vi "Get Users.vi"(8 "error in (no error)":errorcluster, 11 "Data.PG":refnum<class "Data.PGSQL.lvclass">) -> (0 "error out":errorcluster, 2 "Users":string[](array[string]), 3 "Data.PG out":refnum<class "Data.PGSQL.lvclass">)   [LabVIEW 2013, in "Data.PGSQL.lvclass"]
uses:
  Data.PGSQL.lvclass
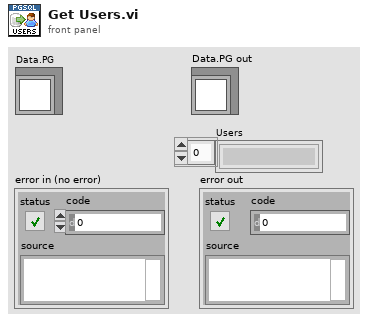
[diagram p1: front panel]
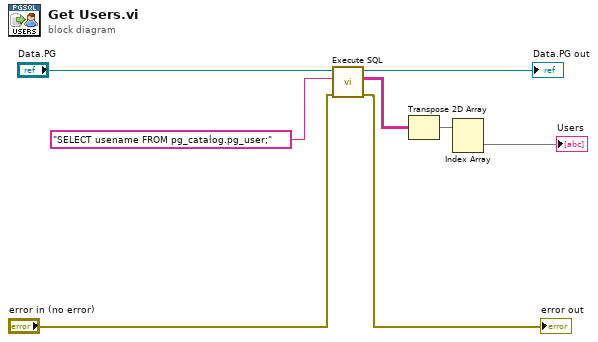
[diagram p0: block diagram]
diagram:
  n1 = call "Execute SQL.vi"("error in"="error in (no error)", "SQL"="SELECT usename FROM pg_catalog.pg_user;" ("command"), "Data.PG"="Data.PG") -> ("error out"=→"error out":errorcluster, "Result"=w5:string[][], "Data.PG out"=→"Data.PG out":refnum<class "Data.PGSQL.lvclass">)  [unwired: 6 in]
  n2 = Transpose 2D Array(2D array=w5) -> (transposed array=w4:string[][])
  n3 = Index Array(array=w4) -> (element=→"Users":string[])  [unwired: 2 in]
